vi "CC.vi"(10 "AD":T2={"电压最大值"=10013, " 电压最小值"=10013, " 采样率"=10013, "每通道采样率"=10013, "采样模式"=10123, "接线方式"=10106, "source"="OnboardClock", "选择通道AD "="USB_6211_2/ai1"} {"采样模式" items=["有限采样"=10178, "连续采样"=10123, "硬件定时单点"=12522]; "接线方式" items=["默认"=-1, "RSE"=10083, "NRSE"=10078, "差分"=10106, "伪差分"=12529]}, 11 "DA":T1={"电压最大值"=0.0, " 电压最小值"=0.0, "选择通道DA "="USB_6211_2/ao1"}) -> (0 "error out":errorcluster caption="错误输出", 3 "prodatascan":T3)   [LabVIEW 2018]
uses:
  Setting/AD.ctl
  Setting/DA.ctl
  ProData/prodatascan.ctl
  <vilib>/DAQmx/read.llb/DAQmx Read (Analog 1D DBL 1Chan NSamp).vi
  <vilib>/DAQmx/read.llb/DAQmx Read (Analog Wfm 1Chan NSamp).vi
  <vilib>/DAQmx/write.llb/DAQmx Write (Analog DBL 1Chan 1Samp).vi
  <vilib>/DAQmx/create/channels.llb/DAQmx Create Channel (AI-Voltage-Basic).vi
  <vilib>/DAQmx/configure/timing.llb/DAQmx Timing (Sample Clock).vi
  <vilib>/DAQmx/miscellaneous.llb/DAQmx Fill In Error Info.vi
  <vilib>/DAQmx/create/channels.llb/DAQmx Create Channel (AO-Voltage-Basic).vi
panel:
  out "AD6211":tag
  out "nVpai":dbl
  out "minindex":i32
  out "maxindex":i32
  out "min":dbl
  out "max":dbl
  out "ScanOut":dbl(graph)
  out "while get stop":bool
  in  "freeCounter":i32=500
  out "free":dbl(graph)
  in  "扫描步进值":dbl=0.005
  out "扫描数据量":dbl
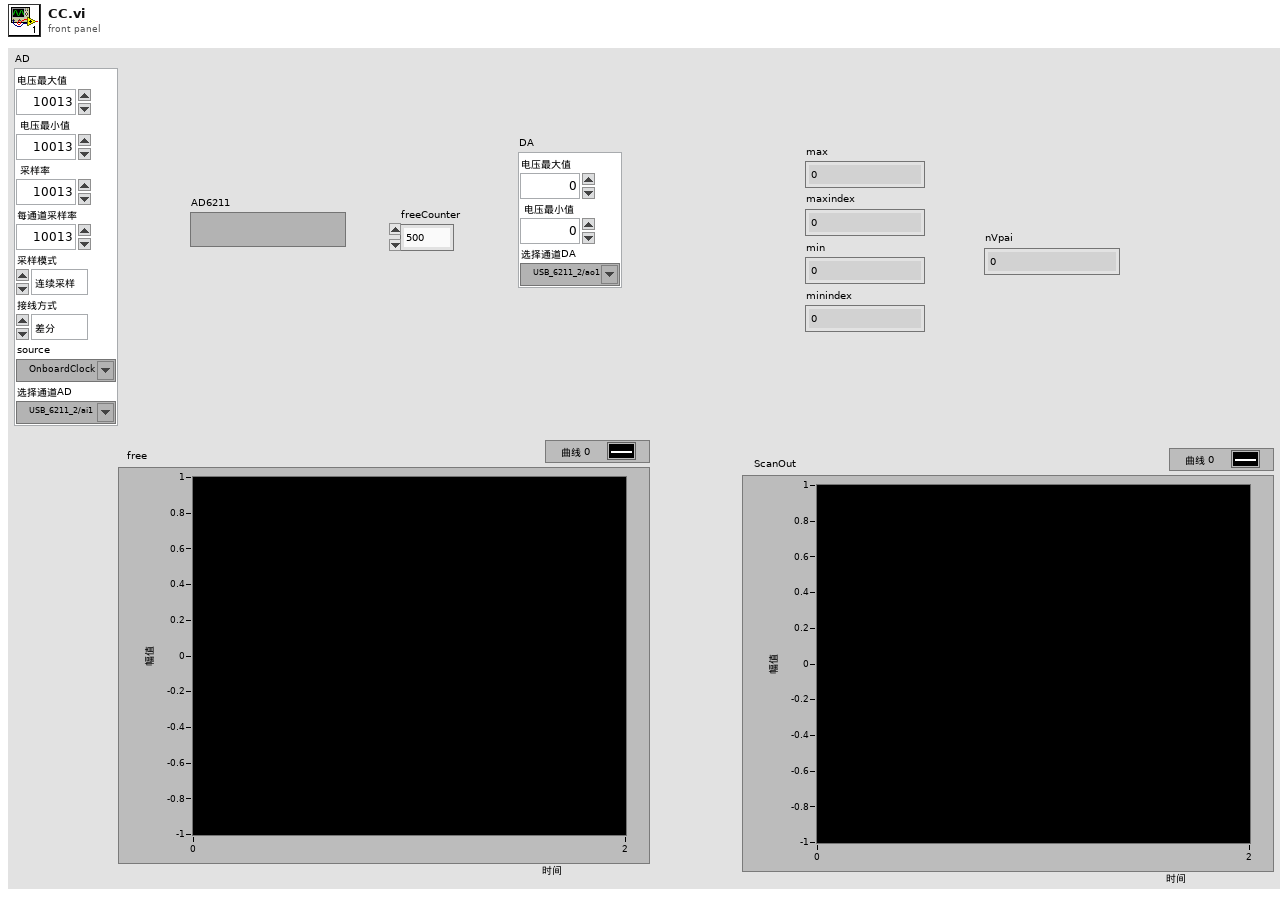
[diagram p1: front panel]
types:
  T1 = typedef "DA.ctl" = cluster{"电压最大值":dbl, " 电压最小值":dbl, "选择通道DA ":tag}
  T2 = typedef "AD.ctl" = cluster{"电压最大值":u16, " 电压最小值":i16, " 采样率":u16, "每通道采样率":u16, "采样模式":i32, "接线方式":i32, "source":tag, "选择通道AD ":tag}
  T3 = cluster{"max":dbl, "min":dbl, " nvpai":dbl, "初始化数组":dbl[]}
  T4 = typedef "prodatascan.ctl" = cluster{"max":dbl, "min":dbl, " nvpai":dbl, "初始化数组":dbl[]}
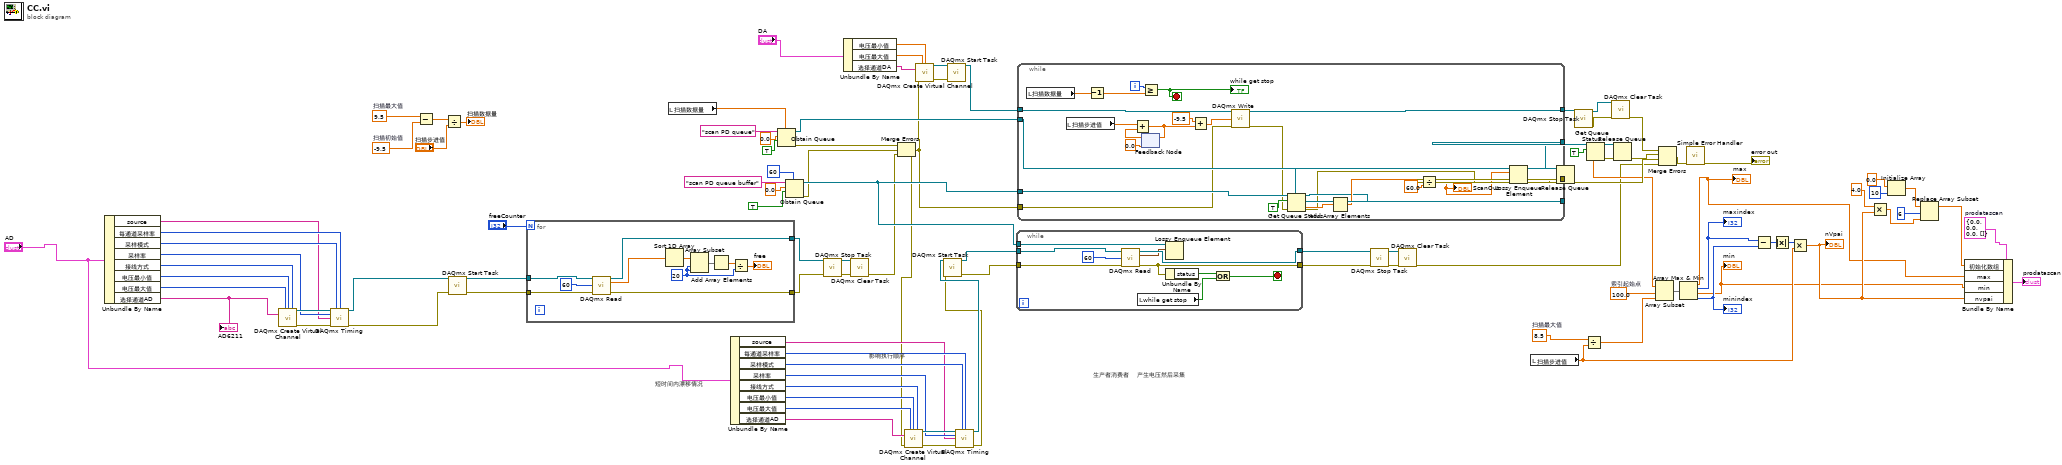
[diagram p0: block diagram]
diagram:
  w24 = T4 {"max"=0.0, "min"=0.0, " nvpai"=0.0, "初始化数组"=[]}  # prodatascan
  w59 = 100.0  # 索引起始点
  w58 = 8.5  # 扫描最大值
  w99 = 9.5  # 扫描最大值
  w100 = -9.5  # 扫描初始值
  # "生产者消费者    产生电压然后采集"
  # "影响执行顺序"
  # "短时间内漂移情况"
  n1 = Unbundle By Name("AD") -> ("source"=w41:tag, "每通道采样率"=w42:u16, "采样模式"=w43:i32, "采样率"=w44:u16, "接线方式"=w50:i32, "电压最小值"=w45:i16, "电压最大值"=w46:u16, "选择通道AD"=w47:tag)
  "AD6211" <- w47
  n2 = call-poly <vilib>:"DAQmx Create Virtual Channel.vi"("maximum value"=w46, "minimum value"=w45, "input terminal configuration"=w50, "physical channels"=w47) -> ("task out"=w49:refnum<k21>, "error out"=w48:errorcluster)  [unwired: 10 in]
  n3 = call-poly <vilib>:"DAQmx Timing.vi"("task/channels in"=w49, "sample mode"=w43, "samples per channel"=w42, "rate"=w44, "source"=w41, "error in"=w48) -> ("task out"=w18:refnum<k21>, "error out"=w40:errorcluster)  [unwired: 8 in]
  n4 = Subtract(x=w99, y=w100) -> (x-y=w101:dbl)
  n5 = Divide(x=w101, y="扫描步进值") -> (x/y=→"扫描数据量":dbl)
  n6 = call <vilib>:"DAQmx Start Task.vi"("task/channels in"=w18, "error in"=w40) -> ("task out"=w94:refnum<k21>, "error out"=w95:errorcluster)  [unwired: 12 in]
  n7 = for {
    N: "freeCounter" -> [_]
    tunnel: w94 -> [w106]
    tunnel: w95 -> [w105]
    tunnel: [w104] -> w19
    tunnel: [w103] -> w20
    w111 = 20 ("索引")
    n8 = call-poly <vilib>:"DAQmx Read.vi"("task/channels in"=w106, "number of samples per channel"=60, "error in"=w105) -> ("task out"=w104:refnum<k21>, "data"=w107:dbl[], "error out"=w103:errorcluster)  [unwired: 10 in]
    n9 = Sort 1D Array(array=w107) -> (sorted array=w112:dbl[])
    n10 = Array Subset(array=w112, index=w111, length=w111) -> (w110:dbl[])
    n11 = Add Array Elements(numeric array=w110) -> (sum=w109:dbl)
    n12 = Divide(x=w109, y=w111) -> (x/y=→"free":dbl)
  }
  n13 = local read "扫描数据量"() -> (w80:dbl)
  n14 = Unbundle By Name("AD") -> ("source"=w8:tag, "每通道采样率"=w9:u16, "采样模式"=w10:i32, "采样率"=w11:u16, "接线方式"=w17:i32, "电压最小值"=w12:i16, "电压最大值"=w13:u16, "选择通道AD"=w14:tag)
  n15 = Obtain Queue(max queue size (-1, unlimited)=w80, name (unnamed)="scan PD queue" ("名称（未命名）"), element data type=0.0, create if not found? (T)=TRUE ("如未找到则创建？(T)")) -> (queue out=w77:refnum<queue>, error out=w75:errorcluster)  [unwired: 1 in, 1 out]
  n16 = Obtain Queue(max queue size (-1, unlimited)=60 ("队列最大值（-1，无限）"), name (unnamed)="scan PD queue buffer" ("名称（未命名）"), element data type=0.0, create if not found? (T)=TRUE ("如未找到则创建？(T)")) -> (queue out=w79:refnum<queue>, error out=w76:errorcluster)  [unwired: 1 in, 1 out]
  n17 = call <vilib>:"DAQmx Stop Task.vi"("task/channels in"=w19, "error in"=w20) -> ("task out"=w3:refnum<k21>, "error out"=w2:errorcluster)  [unwired: 12 in]
  n18 = Unbundle By Name("DA") -> ("电压最小值"=w37:dbl, "电压最大值"=w38:dbl, "选择通道DA"=w39:tag)
  n19 = call <vilib>:"DAQmx Clear Task.vi"("task in"=w3, "error in"=w2) -> ("error out"=w1:errorcluster)  [unwired: 13 in]
  n20 = Merge Errors(w75, w76, w1) -> (w5:errorcluster)
  n21 = call-poly <vilib>:"DAQmx Create Virtual Channel.vi"("maximum value"=w13, "minimum value"=w12, "input terminal configuration"=w17, "physical channels"=w14, "error in"=w5) -> ("task out"=w16:refnum<k21>, "error out"=w15:errorcluster)  [unwired: 9 in]
  n22 = call-poly <vilib>:"DAQmx Create Virtual Channel.vi"("maximum value"=w38, "minimum value"=w37, "physical channels"=w39, "error in"=w5) -> ("task out"=w86:refnum<k21>, "error out"=w85:errorcluster)  [unwired: 10 in]
  n23 = call <vilib>:"DAQmx Start Task.vi"("task/channels in"=w86, "error in"=w85) -> ("task out"=w78:refnum<k21>)  [unwired: 12 in, 1 out]
  n24 = call-poly <vilib>:"DAQmx Timing.vi"("task/channels in"=w16, "sample mode"=w10, "samples per channel"=w9, "rate"=w11, "source"=w8, "error in"=w15) -> ("task out"=w6:refnum<k21>, "error out"=w4:errorcluster)  [unwired: 8 in]
  n25 = call <vilib>:"DAQmx Start Task.vi"("task/channels in"=w6, "error in"=w4) -> ("task out"=w22:refnum<k21>, "error out"=w21:errorcluster)  [unwired: 12 in]
  n26 = while {
    tunnel: w21 -> [w122]
    tunnel: [w121] -> w93
    tunnel: [w120] -> w92
    tunnel: w79 -> [w117]
    tunnel: w22 -> [w114]
    stop <- w118 stop-if-true
    n27 = call-poly <vilib>:"DAQmx Read.vi"("task/channels in"=w114, "number of samples per channel"=60, "error in"=w122) -> ("task out"=w121:refnum<k21>, "data"=w116:waveform(dbl), "error out"=w120:errorcluster)  [unwired: 10 in]
    n28 = local read "while get stop"() -> (w113:bool)
    n29 = Lossy Enqueue Element(queue=w117, element=w116) -> ()  [unwired: 1 in, 4 out]
    n30 = Unbundle By Name(w120) -> ("status"=w119:bool)
    n31 = Or(x=w119, y=w113) -> (x .or. y?=w118:bool)
  }
  n32 = while {
    tunnel: w79 -> [w128]
    tunnel: w78 -> [w147]
    tunnel: w77 -> [w129]
    tunnel: w5 -> [w123]
    tunnel: [w131] -> w72
    tunnel: [w130] -> w71
    tunnel: [w127] -> w56
    tunnel: [w126] -> w52
    i -> [w138]
    stop <- w137 stop-if-true
    n33 = local read "扫描数据量"() -> (w140:dbl)
    n34 = local read "扫描步进值"() -> (w146:dbl)
    n35 = Decrement(x=w140) -> (x-1=w139:dbl)
    n36 = feedback #1(0.0) -> (w144:dbl)
    n37 = Add(x=w146, y=w144) -> (x+y=w143:dbl)
    n38 = feedback-in #1(w143) -> ()
    n39 = Greater Or Equal?(x=w138, y=w139) -> (x >= y?=w137:bool)
    "while get stop" <- w137
    n40 = Add(x=-9.5, y=w143) -> (x+y=w141:dbl)
    n41 = call-poly <vilib>:"DAQmx Write.vi"("task/channels in"=w147, "data"=w141, "error in"=w123) -> ("task out"=w131:refnum<k21>, "error out"=w125:errorcluster)  [unwired: 10 in, 1 out]
    n42 = Get Queue Status(queue=w128, return elements? (F)=TRUE ("返回元素？(F)"), error in (no error)=w125) -> (queue out=w126:refnum<queue>, error out=w124:errorcluster, elements=w135:dbl[])  [unwired: 5 out]
    n43 = Add Array Elements(numeric array=w135) -> (sum=w134:dbl)
    n44 = Divide(x=w134, y=60.0) -> (x/y=w132:dbl)
    "ScanOut" <- w132
    n45 = Lossy Enqueue Element(queue=w129, element=w132, error in (no error)=w124) -> (queue out=w127:refnum<queue>, error out=w130:errorcluster)  [unwired: 2 out]
  }
  n46 = call <vilib>:"DAQmx Stop Task.vi"("task/channels in"=w93, "error in"=w92) -> ("task out"=w90:refnum<k21>, "error out"=w91:errorcluster)  [unwired: 12 in]
  n47 = call <vilib>:"DAQmx Clear Task.vi"("task in"=w90, "error in"=w91) -> ("error out"=w51:errorcluster)  [unwired: 13 in]
  n48 = local read "扫描步进值"() -> (w57:dbl)
  n49 = Release Queue(queue=w52, error in (no error)=w71) -> (error out=w69:errorcluster)  [unwired: 1 in, 2 out]
  n50 = call <vilib>:"DAQmx Stop Task.vi"("task/channels in"=w72) -> ("task out"=w74:refnum<k21>, "error out"=w73:errorcluster)  [unwired: 13 in]
  n51 = Divide(x=w58, y=w57) -> (x/y=w65:dbl)
  n52 = Get Queue Status(queue=w56, return elements? (F)=TRUE ("返回元素？(F)")) -> (queue out=w53:refnum<queue>, error out=w55:errorcluster, elements=w66:dbl[])  [unwired: 1 in, 5 out]
  n53 = call <vilib>:"DAQmx Clear Task.vi"("task in"=w74, "error in"=w73) -> ("error out"=w70:errorcluster)  [unwired: 13 in]
  n54 = Release Queue(queue=w53, error in (no error)=w55) -> (error out=w54:errorcluster)  [unwired: 1 in, 2 out]
  n55 = Array Subset(array=w66, index=w59, length=w65) -> (w64:dbl[])
  n56 = Merge Errors(w70, w54, w69, w51) -> (w68:errorcluster)
  n57 = Array Max & Min(array=w64) -> (max value=w28:dbl, max index (indices)=w60:i32, min value=w27:dbl, min index (indices)=w63:i32)
  "max" <- w28
  "min" <- w27
  "maxindex" <- w60
  "minindex" <- w63
  n58 = call <vilib>:"Simple Error Handler.vi"("error in (no error)"=w68) -> ("error out"=→"error out":errorcluster)  [unwired: 4 in, 4 out]
  n59 = Subtract(x=w60, y=w63) -> (x-y=w62:i32)
  n60 = Absolute Value(x=w62) -> (abs(x)=w61:i32)
  n61 = Multiply(x=w61, y=w57) -> (x*y=w29:dbl)
  "nVpai" <- w29
  n62 = Multiply(x=4.0, y=w29) -> (x*y=w32:dbl)
  n63 = Initialize Array(0.0 ("元素"), 10 ("维数大小")) -> (w34:dbl[])
  n64 = Replace Array Subset(array=w34, new element=w32, index=6 ("索引")) -> (w31:dbl[])
  n65 = Bundle By Name(cluster=w24, "初始化数组"=w31, "max"=w28, "min"=w27, "nvpai"=w29) -> (→"prodatascan":T4)
